vi "setReadFIFO.vi"(10 "IReadFIFO":refnum<class "IReadFIFO.lvclass">, 11 "RTHealthAndStatus in":refnum<class "RTHealthAndStatus.lvclass">) -> (3 "RTHealthAndStatus out":refnum<class "RTHealthAndStatus.lvclass">)   [LabVIEW 2015, in "RTHealthAndStatus.lvlib" / "RTHealthAndStatus.lvclass"]
uses:
  RTHealthAndStatus.lvclass
  Common_RT_FPGA/IReadFIFO/IReadFIFO.lvclass
  RTHealthAndStatus.lvclass/RTHealthAndStatus.ctl
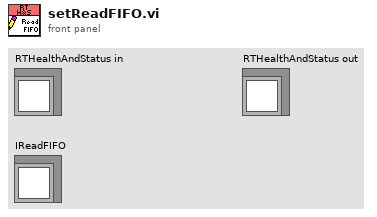
[diagram p1: front panel]
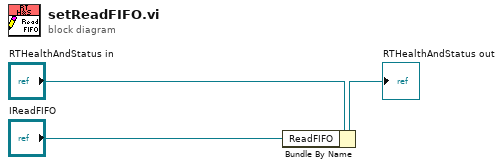
[diagram p0: block diagram]
diagram:
  n1 = Bundle By Name(cluster="RTHealthAndStatus in", "ReadFIFO"="IReadFIFO") -> (→"RTHealthAndStatus out":refnum<class "RTHealthAndStatus.lvclass">)
